vi "15.-Lectura de Señal, Creación de Tablas y Almacenamiento en un Archivo.vi"() -> ()   [LabVIEW 2020]
uses:
  <vilib>/Utility/file.llb/Write Delimited Spreadsheet (DBL).vi
  <vilib>/Analysis/NI_AALBase.lvlib
panel:
  out "Table Control":string[][](table)
  out "Waveform Graph":dbl[][](graph)
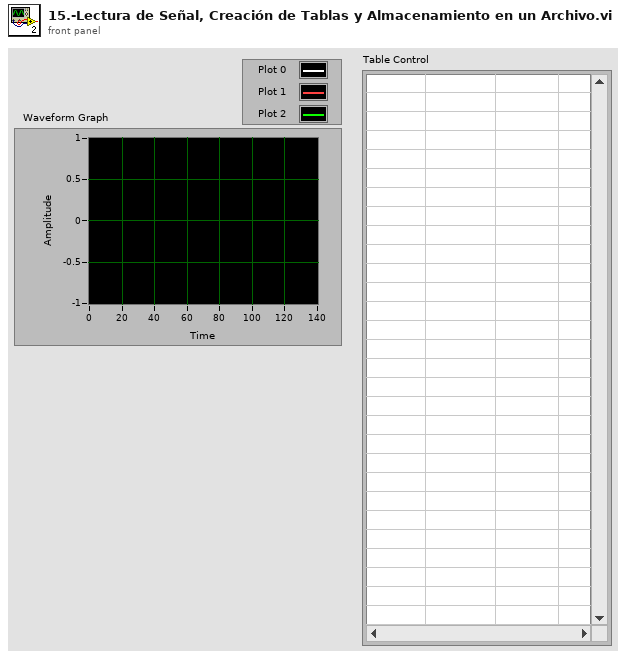
[diagram p1: front panel]
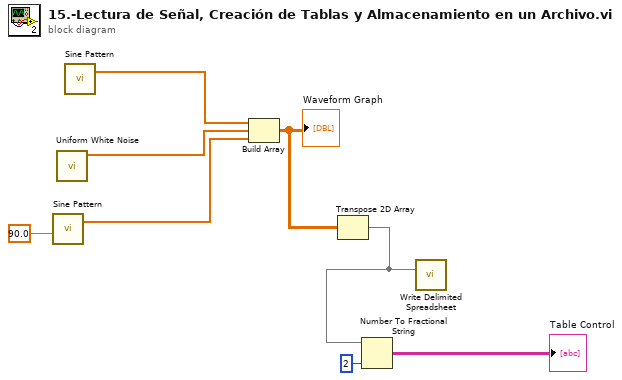
[diagram p0: block diagram]
diagram:
  n1 = call <vilib>:"Sine Pattern.vi"("phase(degrees)"=90.0) -> ("Sinusoidal Pattern"=w6:dbl[])  [unwired: 3 in, 1 out]
  n2 = call <vilib>:"Uniform White Noise.vi"() -> ("uniform white noise"=w7:dbl[])  [unwired: 10 in, 1 out]
  n3 = call <vilib>:"Sine Pattern.vi"() -> ("Sinusoidal Pattern"=w8:dbl[])  [unwired: 4 in, 1 out]
  n4 = Build Array(w8, w7, w6) -> (w4:dbl[][])
  "Waveform Graph" <- w4
  n5 = Transpose 2D Array(2D array=w4) -> (transposed array=w3:dbl[][])
  n6 = Number To Fractional String(number=w3, precision (6)=i16 2) -> (F-format string=→"Table Control":string[][])  [unwired: 2 in]
  n7 = call-poly <vilib>:"Write Delimited Spreadsheet.vi"("2D data"=w3) -> ()  [unwired: 13 in, 2 out]
